vi "UART_W&R.vi"(4 "Add Return":bool=TRUE, 5 "ExpectStr":string="OK", 6 "error in (no error)":errorcluster, 7 "Delay (s)":dbl=0.1 caption="Delay Time (s)", 8 "write buffer":string=">01 DOWNLOAD", 9 "FIX_COM":refnum<visa-resource-name>="COM1") -> (0 "error out":errorcluster, 1 "OK?":bool, 2 "StrOut":string, 3 "VISA Resource Out":refnum<visa-resource-name>)   [LabVIEW 2011]
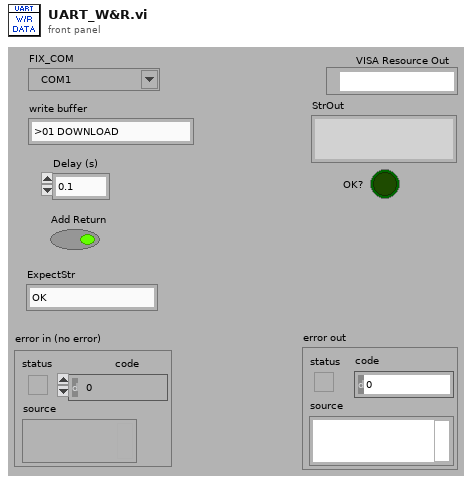
[diagram p1: front panel]
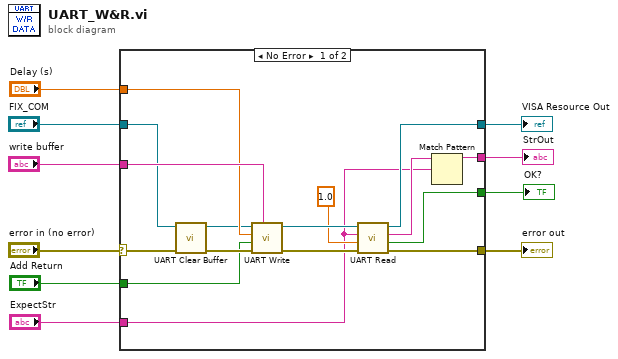
[diagram p0: block diagram]
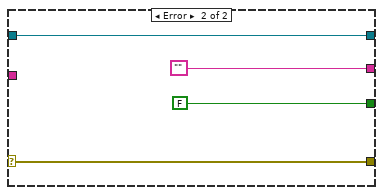
[diagram p2: hidden frame]
diagram:
  n1 = case shown="No Error" "error in (no error)" {
    selector: "error in (no error)" -> [w19 w29]
    tunnel: "FIX_COM" -> [w17 w30]
    tunnel: [w22 w29] -> w5
    tunnel: [w21 w30] -> w9
    tunnel: "write buffer" -> [w26 _]
    tunnel: "Delay (s)" -> [w25 _]
    tunnel: [w13 ""] -> w4
    tunnel: [w15 FALSE ("OK?")] -> w3
    tunnel: "ExpectStr" -> [w12 _]
    tunnel: "Add Return" -> [w11 _]
    frame No Error {
      n2 = call "UART Clear Buffer.vi"("Error In"=w19, "VISA Resource In"=w17) -> ("Error Out"=w18:errorcluster, "VISA Resource Out"=w16:refnum<visa-resource-name>)  [unwired: 5 in]
      n3 = call "UART Write.vi"("write buffer"=w26, "error in (no error)"=w18, "Add Return"=w11, "Write Delay (s)"=w25, "VISA Resource In"=w16) -> ("error out"=w24:errorcluster, "VISA Resource Out"=w23:refnum<visa-resource-name>)  [unwired: 2 in]
      n4 = call "UART Read.vi"("error in (no error)"=w24, "TimeOut(s)"=1.0, "ExpectStr"=w12, "VISA Resource In"=w23) -> ("error out"=w22:errorcluster, "OK?"=w15:bool, "StrOut"=w14:string, "VISA Resource Out"=w21:refnum<visa-resource-name>)  [unwired: 1 in]
      n5 = Match Pattern(string=w14, regular expression=w12) -> (before substring=w13:string)  [unwired: 1 in, 3 out]
    }
    frame Error {
    }
  }
  "error out" <- w5
  "VISA Resource Out" <- w9
  "StrOut" <- w4
  "OK?" <- w3
